vi "NanonisProperties_FBL.vi"(0 "Application reference":refnum<vi>, 1 "Z Write (m)":sgl format="%#_6p", 5 "X pen (nm)":dbl, 7 "Z pen (nm)":dbl, 11 "Error in":errorcluster, 12 "Z Write?":bool) -> (2 "Frame Size (m)":cluster{"Width":sgl, "Height":sgl} {"Height" format="%.2p"; "Width" format="%.2p"}, 3 "Frame Origin (m)":cluster{"Xc":sgl, "Yc":sgl} {"Yc" format="%.2p"; "Xc" format="%.2p"}, 4 "Application ref out":refnum<vi>, 6 "Setpoint (pA)":sgl format="%#_6p", 8 "Current (pA)":sgl format="%#_6p", 10 "Z Read (m)":sgl format="%#_6p", 15 "error out":errorcluster)   [LabVIEW 2019]
uses:
  <userlib>/Nanonis Prog Interface V5/Nanonis Prog Interface.lvlib
panel:
  out "prog int?":bool
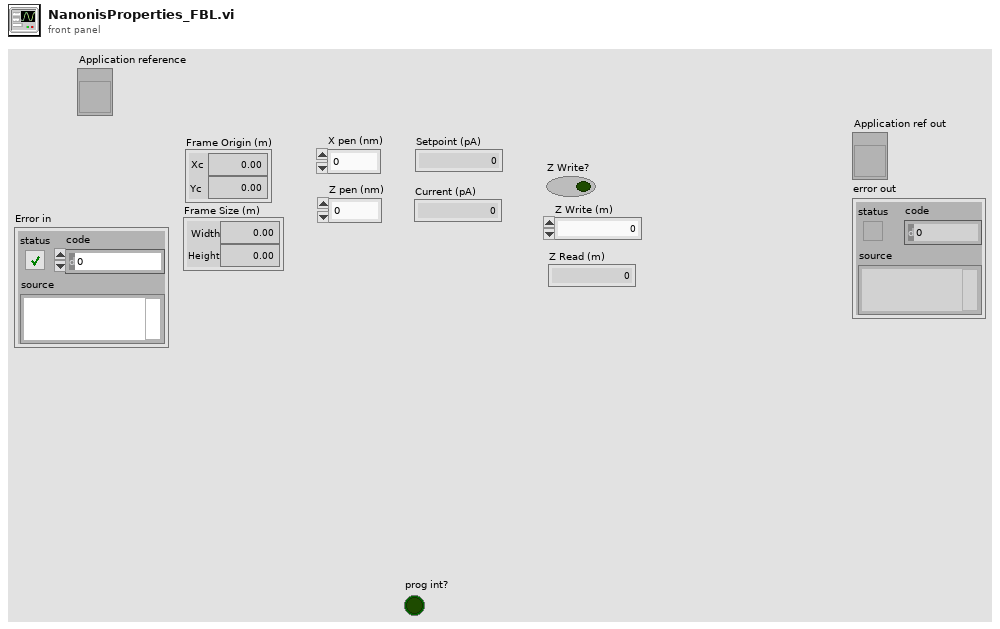
[diagram p1: front panel]
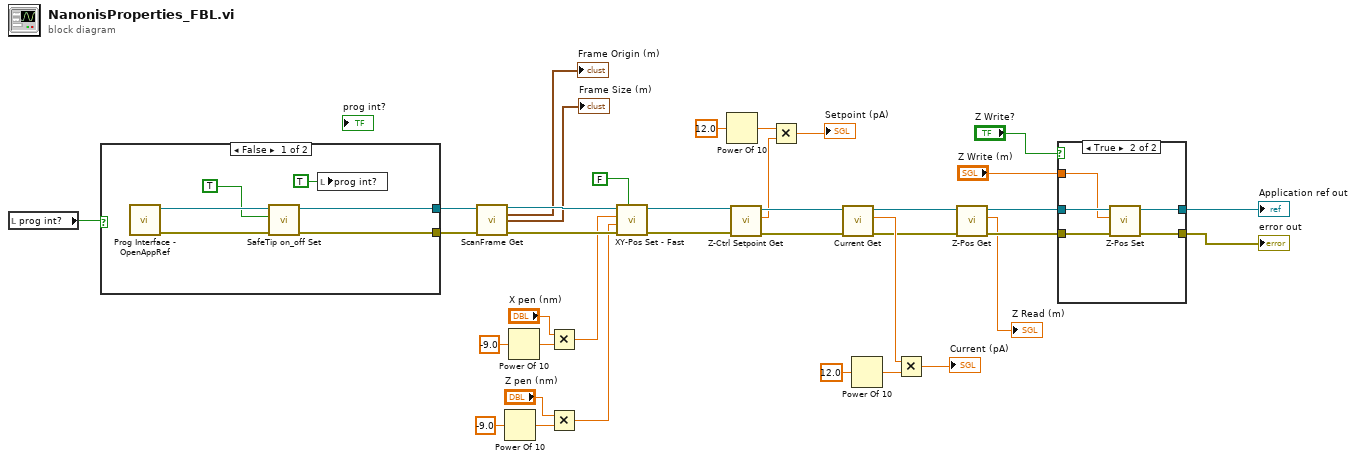
[diagram p0: block diagram]
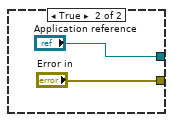
[diagram p3: hidden frame]
diagram:
  n1 = local read "prog int?"() -> (w1:bool)
  n2 = case shown="False" w1 {
    tunnel: [w39 "Application reference"] -> w36
    tunnel: [w38 "Error in"] -> w35
    frame False {
      n3 = call <userlib>:"Prog Interface - OpenAppRef.vi"() -> ("Error out"=w42:errorcluster, "Application reference"=w41:refnum<vi>)  [unwired: 6 in]
      n4 = call <userlib>:"SafeTip on_off Set.vi"("error in (no error)"=w42, "SafeTip ON/OFF"=TRUE, "Application ref in"=w41) -> ("error out"=w38:errorcluster, "Application ref out"=w39:refnum<vi>)  [unwired: 7 in]
      n5 = local write "prog int?"(TRUE ("prog int?")) -> ()
    }
    frame True {
    }
  }
  n6 = call <userlib>:"ScanFrame Get.vi"("Application ref in"=w36, "error in (no error)"=w35) -> ("Application ref out"=w34:refnum<vi>, "Center coordinates (m)"=→"Frame Origin (m)":cluster{"Xc":sgl, "Yc":sgl}, "Size (m)"=→"Frame Size (m)":cluster{"Width":sgl, "Height":sgl}, "error out"=w33:errorcluster)  [unwired: 9 in, 1 out]
  n7 = Power Of 10(x=-9.0) -> (10^x=w27:dbl)
  n8 = Power Of 10(x=-9.0) -> (10^x=w30:dbl)
  n9 = Multiply(x="X pen (nm)", y=w30) -> (x*y=w24:dbl)
  n10 = Multiply(x="Z pen (nm)", y=w27) -> (x*y=w23:dbl)
  n11 = call <userlib>:"XY-Pos Set - Fast.vi"("Wait end-of-motion (T=True)"=FALSE, "error in (no error)"=w33, "Y (m)"=w23, "X (m)"=w24, "Application ref in"=w34) -> ("error out"=w17:errorcluster, "Application ref out"=w18:refnum<vi>)  [unwired: 4 in]
  n12 = Power Of 10(x=12.0) -> (10^x=w12:dbl)
  n13 = call <userlib>:"Z-Ctrl Setpoint Get.vi"("error in (no error)"=w17, "Application ref in"=w18) -> ("error out"=w15:errorcluster, "Z Controller setpoint"=w11:sgl, "Application ref out"=w16:refnum<vi>)  [unwired: 6 in]
  n14 = Multiply(x=w12, y=w11) -> (x*y=→"Setpoint (pA)":dbl)
  n15 = call <userlib>:"Current Get.vi"("Error in (no error)"=w15, "Application ref in"=w16) -> ("Error out"=w9:errorcluster, "Current (A)"=w19:sgl, "Application ref out"=w10:refnum<vi>)  [unwired: 5 in]
  n16 = Power Of 10(x=12.0) -> (10^x=w20:dbl)
  n17 = Multiply(x=w19, y=w20) -> (x*y=→"Current (pA)":dbl)
  n18 = call <userlib>:"Z-Pos Get.vi"("error in (no error)"=w9, "Application ref in"=w10) -> ("error out"=w7:errorcluster, "Z position (m)"=→"Z Read (m)":sgl, "Application ref out"=w8:refnum<vi>)  [unwired: 7 in]
  n19 = case shown="True" "Z Write?" {
    tunnel: w8 -> [w47 w52]
    tunnel: w7 -> [w46 w51]
    tunnel: [w47 w50] -> w6
    tunnel: [w46 w49] -> w5
    tunnel: "Z Write (m)" -> [_ w48]
    frame False {
    }
    frame True {
      n20 = call <userlib>:"Z-Pos Set.vi"("error in (no error)"=w51, "Z position (m)"=w48, "Application ref in"=w52) -> ("error out"=w49:errorcluster, "Application ref out"=w50:refnum<vi>)  [unwired: 7 in]
    }
  }
  "Application ref out" <- w6
  "error out" <- w5
